vi "Get new anlge to rotate filter wheel by.vi"(9 "Filter Wheel Positions":dbl[][](array[numeric])=[[0.0, 0.0], [1.0, 30.0], [2.0, 60.0], [3.0, 90.0], [4.0, 120.0], [5.0, 150.0], [6.0, 180.0], [7.0, 210.0], [8.0, 240.0], [9.0, 270.0], [10.0, 300.0], [11.0, 336.5]], 10 "Current anlge (degrees)":dbl, 11 "Filter no.":dbl) -> (0 "Clockwise?":bool, 3 "Rotate by angle (degrees)":dbl, 4 "New current anlge (degrees)":dbl)   [LabVIEW 2011]
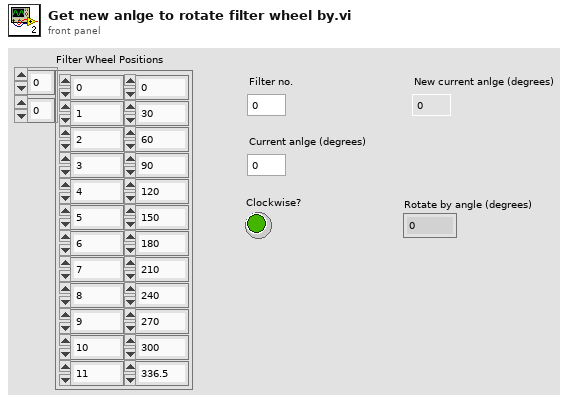
[diagram p1: front panel]
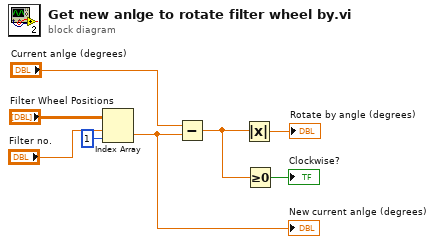
[diagram p0: block diagram]
diagram:
  n1 = Index Array(array="Filter Wheel Positions", index (row)="Filter no.", index (col)=1 ("disabled index (col)")) -> (element=w1:dbl)
  "New current anlge (degrees)" <- w1
  n2 = Subtract(x="Current anlge (degrees)", y=w1) -> (x-y=w3:dbl)
  n3 = Absolute Value(x=w3) -> (abs(x)=→"Rotate by angle (degrees)":dbl)
  n4 = Greater Or Equal To 0?(x=w3) -> (x >= 0?=→"Clockwise?":bool)
